vi "physics lab 2.vi"() -> ()   [LabVIEW 2019]
panel:
  out "error out":errorcluster
  in  "error in (no error)":errorcluster
  out "Time to update (ms)":dbl
  out "Waveform Chart":dbl(graph)
  in  "speed":dbl(knob)=1000.0 scale=0.0..1000.0
  in  "stop":bool
  in  "N":i32
  out "Alarm":bool
  in  "F0":dbl
  in  "x0":dbl(slide) scale=-3.0..3.0
  in  "m":dbl
  in  "dt":dbl
  in  "k":dbl
  in  "b":dbl
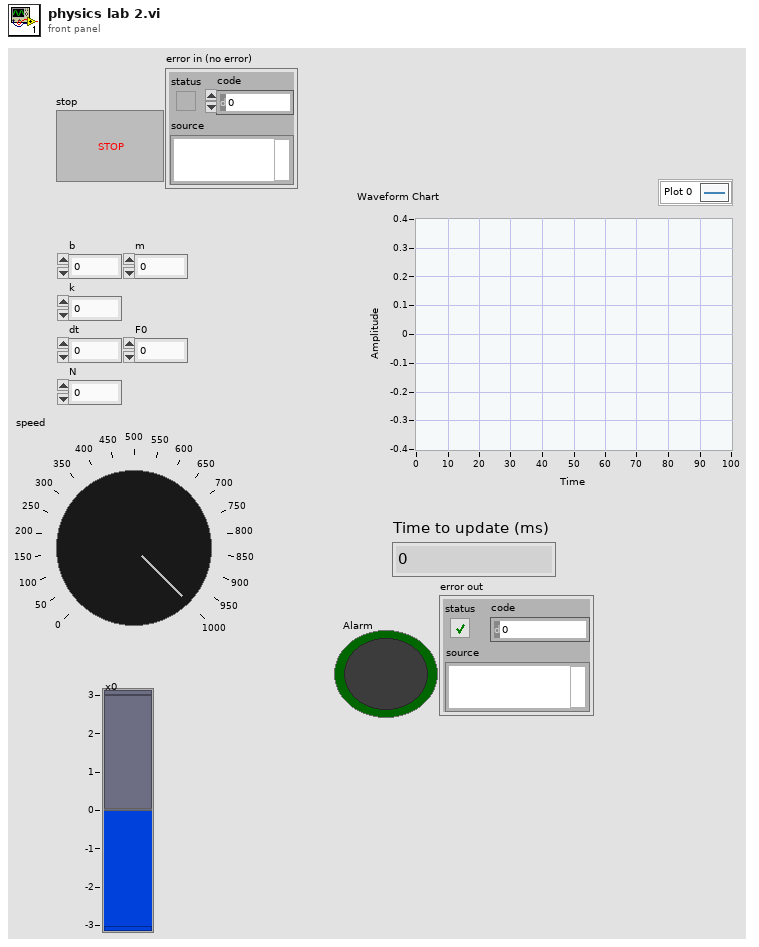
[diagram p1: front panel]
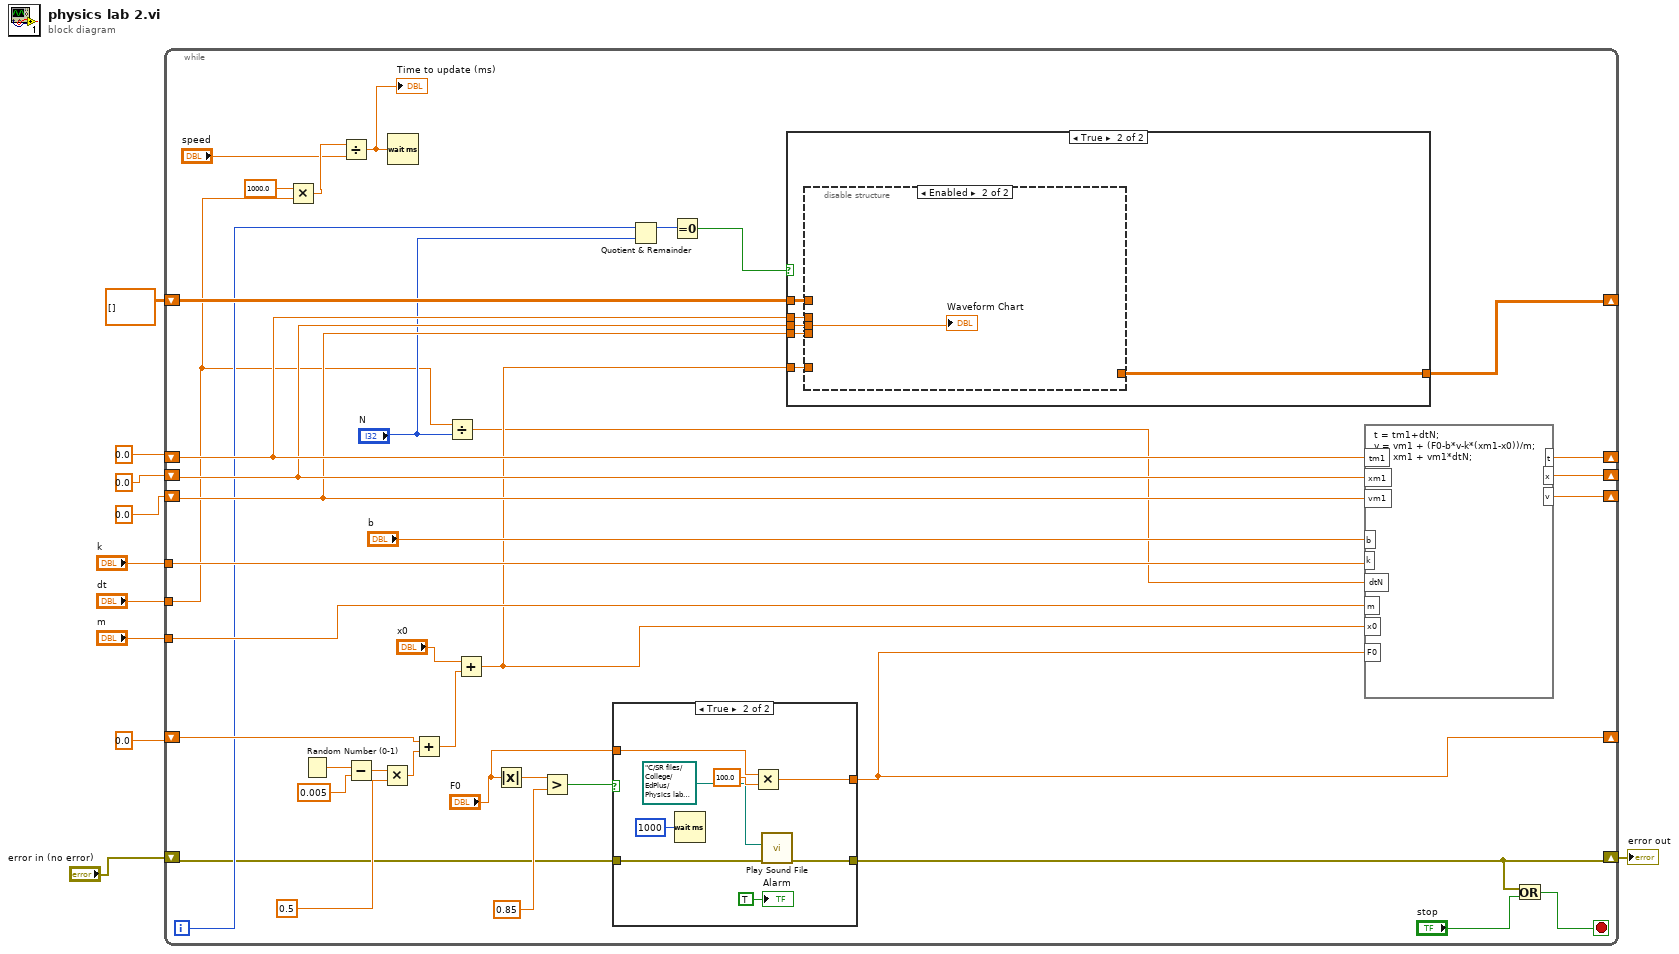
[diagram p0: block diagram]
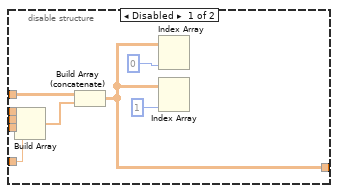
[diagram p3: hidden frame]
diagram:
  n1 = while {
    tunnel: "k" -> [w48]
    tunnel: "dt" -> [w19]
    tunnel: "m" -> [w47]
    shift-right: [w34] -> _
    shift-left: 0.0 -> [w30]
    shift-right: [w33] -> _
    shift-left: 0.0 -> [w29]
    shift-right: [w32] -> _
    shift-left: 0.0 -> [w28]
    shift-right: [w31] -> _
    shift-left: 0.0 -> [w46]
    shift-right: [w26] -> _
    shift-left: dbl[][] [] -> [w25]
    shift-right: [w13] -> w2
    shift-left: "error in (no error)" -> [w11]
    i -> [w24]
    stop <- w12 stop-if-true
    n2 = Multiply(x=1000.0, y=w19) -> (x*y=w17:dbl)
    n3 = Random Number (0-1)() -> (number: 0 to 1=w43:dbl)
    n4 = Divide(x=w17, y="speed") -> (x/y=w15:dbl)
    "Time to update (ms)" <- w15
    n5 = Subtract(x=w43, y=0.005) -> (x-y=w44:dbl)
    n6 = Multiply(x=w44, y=0.5) -> (x*y=w45:dbl)
    n7 = Wait (ms)(milliseconds to wait=w15) -> ()  [unwired: 1 out]
    n8 = Add(x=w46, y=w45) -> (x+y=w36:dbl)
    n9 = Divide(x=w19, y="N") -> (x/y=w23:dbl)
    n10 = Add(x="x0", y=w36) -> (x+y=w27:dbl)
    n11 = Absolute Value(x="F0") -> (abs(x)=w39:dbl)
    n12 = Greater?(x=w39, y=0.85) -> (0:w37:bool)
    n13 = case shown="True" w37 {
      tunnel: "F0" -> [w68 w76]
      tunnel: [w68 w71] -> w31
      tunnel: w11 -> [w67 w70]
      tunnel: [w67 w69] -> w13
      frame False {
      }
      frame True {
        n14 = Wait (ms)(milliseconds to wait=u32 1000) -> ()  [unwired: 1 out]
        n15 = Multiply(x=w76, y=100.0) -> (x*y=w71:dbl)
        n16 = call <vilib>:"Play Sound File.vi"("error in (no error)"=w70, "path"=path "C:/SR files/College/EdPlus/Physics lab project/LabVIEW/alarm2.mp3") -> ("error out"=w69:errorcluster)  [unwired: 8 in, 1 out]
        "Alarm" <- TRUE ("Alarm")
      }
    }
    n17 = Quotient & Remainder(x=w24, y="N") -> (x-y*floor(x/y)=w21:i32)  [unwired: 1 out]
    n18 = Equal To 0?(x=w21) -> (x = 0?=w20:bool)
    n19 = case shown="True" w20 {
      tunnel: w30 -> [_ w56]
      tunnel: w29 -> [_ w55]
      tunnel: w28 -> [_ w54]
      tunnel: w27 -> [_ w53]
      tunnel: [w50 w52] -> w26
      tunnel: w25 -> [w50 w51]
      frame False {
      }
      frame True {
        n20 = disable-structure shown="Enabled" {
          disable-tunnel: w56 -> [w65 _]
          disable-tunnel: w55 -> [w64 w66]
          disable-tunnel: w54 -> [w63 _]
          disable-tunnel: w53 -> [w62 _]
          disable-tunnel: [w60 _] -> w52
          disable-tunnel: w51 -> [w59 _]
          frame Disabled {
            n21 = Build Array(w65, w64, w63, w62) -> (w61:dbl[])
            n22 = Build Array (concatenate)(w59, w61) -> (w60:dbl[][])
            n23 = Index Array(array=w60, index (col)=0 ("index (row)")) -> ()  [unwired: 1 in, 1 out]
            n24 = Index Array(array=w60, index (col)=1 ("index (row)")) -> ()  [unwired: 1 in, 1 out]
          }
          frame Enabled {
            "Waveform Chart" <- w66
          }
        }
      }
    }
    n25 = formula code="t = tm1+dtN;\nv = vm1 + (F0-b*v-k*(xm1-x0))/m;\nx = xm1 + vm1*dtN;"("tm1"=w30, "xm1"=w29, "vm1"=w28, "b"="b", "k"=w48, "dtN"=w23, "m"=w47, "x0"=w27, "F0"=w31) -> ("t"=w34:dbl, "x"=w33:dbl, "v"=w32:dbl)
    n26 = Or(x=w13, y="stop") -> (x .or. y?=w12:bool)
  }
  "error out" <- w2
